vi "SignalAnalyzer.vi"() -> ()   [LabVIEW 2020]
uses:
  <vilib>/Analysis/2dsp.llb/Real FFT.vi
  <vilib>/Analysis/NI_AALPro.lvlib
panel:
  out "Waveform Graph 1+2 \nFFT":dbl[](graph)
  out "Waveform Graph 2":dbl[](graph)
  out "Waveform Graph 1":dbl[](graph)
  in  "stop":bool
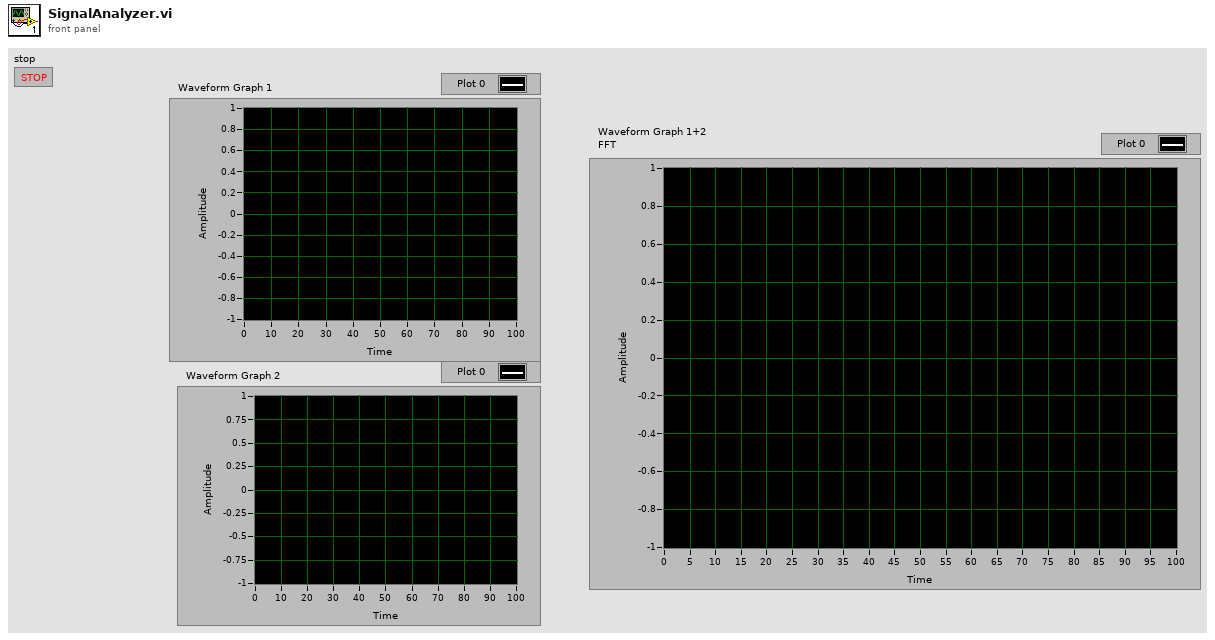
[diagram p1: front panel]
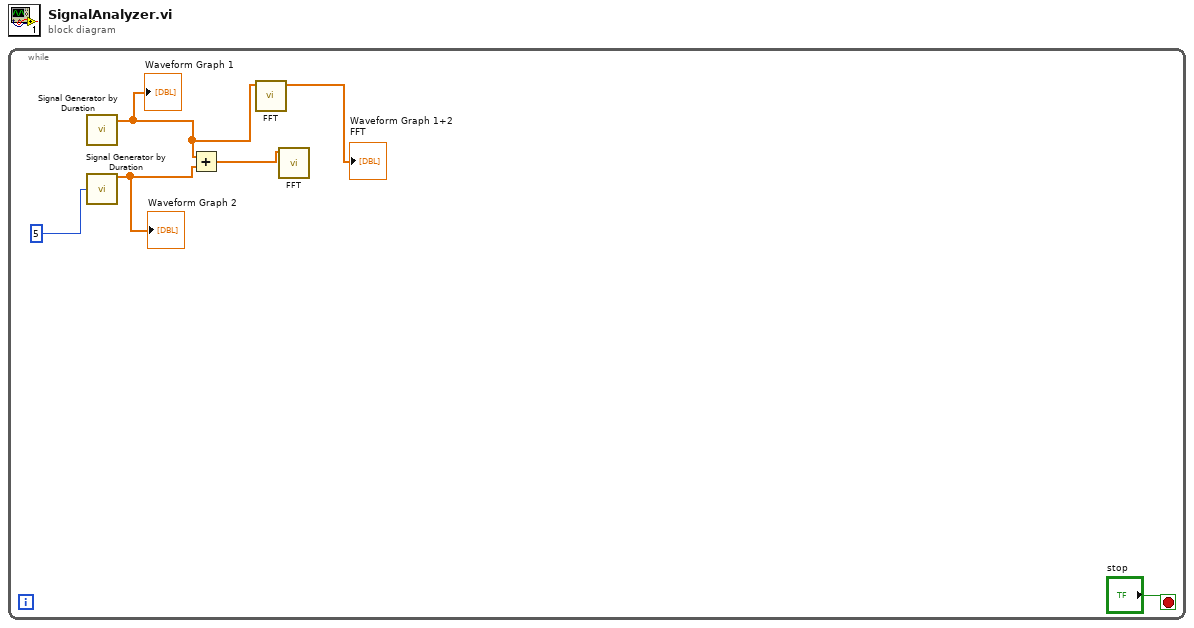
[diagram p0: block diagram]
diagram:
  n1 = while {
    stop <- "stop" stop-if-true
    n2 = call <vilib>:"Signal Generator by Duration.vi"() -> ("signal"=w2:dbl[])  [unwired: 12 in, 3 out]
    "Waveform Graph 1" <- w2
    n3 = call <vilib>:"Signal Generator by Duration.vi"("frequency"=5) -> ("signal"=w4:dbl[])  [unwired: 11 in, 3 out]
    "Waveform Graph 2" <- w4
    n4 = Add(x=w2, y=w4) -> (x+y=w5:dbl[])
    n5 = call-poly <vilib>:"FFT.vi"("X"=w2) -> ("FFT {X}"=→"Waveform Graph 1+2 \nFFT":cdb[])  [unwired: 9 in, 1 out]
    n6 = call-poly <vilib>:"FFT.vi"("X"=w5) -> ()  [unwired: 9 in, 2 out]
  }
